vi "GA E Stop Set IO.vi"(7 "lFilterTime":u32, 8 "error in (no error)":errorcluster caption="错误输入（无错误）", 9 "nEStopSns":i16, 10 "nIOIndex":i16, 11 "nCardIndex":i16) -> (0 "error out":errorcluster caption="错误输出", 3 "function return":i32)   [LabVIEW 2015, in "GAS.lvlib"]
doc: "extern \"C\" __declspec(dllimport) int GA_EStopSetIO(short nCardIndex,short nIOIndex,short nEStopSns,unsigned long lFilterTime);"
uses:
  <userlib>/BP_GAS/GAS.lvlib
  <userlib>/BP_GAS/GAS.dll
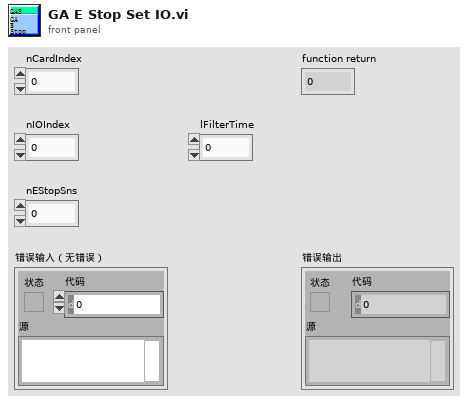
[diagram p1: front panel]
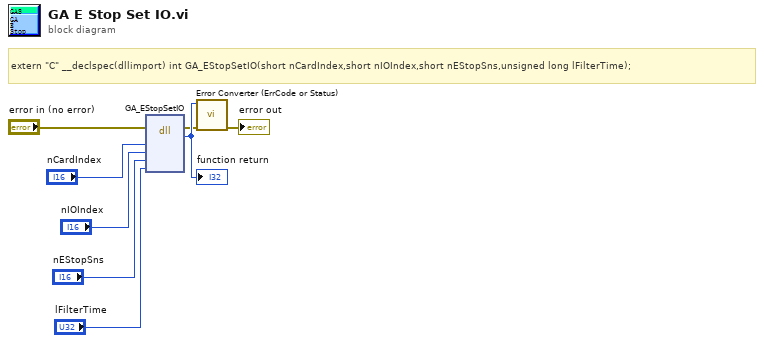
[diagram p0: block diagram]
diagram:
  # "extern \"C\" __declspec(dllimport) int GA_EStopSetIO(short nCardIndex,short nIOIndex,short nEStopSns,unsigned long lFilterTime);"
  n1 = dll-call lib="E:/Program Files (x86)/National Instruments/LabVIEW 2015/user.lib/BP_GAS/GAS.*" fn="GA_EStopSetIO"(error in="error in (no error)", "nCardIndex"="nCardIndex", "nIOIndex"="nIOIndex", "nEStopSns"="nEStopSns", "lFilterTime"="lFilterTime") -> (error out=w2:errorcluster, w8:i32)  [unwired: 6 in, 1 out]
  "function return" <- w8
  n2 = call "Error Converter (ErrCode or Status).vi"("error in (no error)"=w2, "error code"=w8) -> ("error out"=→"error out":errorcluster)  [unwired: 9 in]
